vi "GRAPH.vi"() -> ()   [LabVIEW 2013]
panel:
  in  "Power":i32 min=0 max=100 step=1
  out "Waveform Chart":i32(graph)
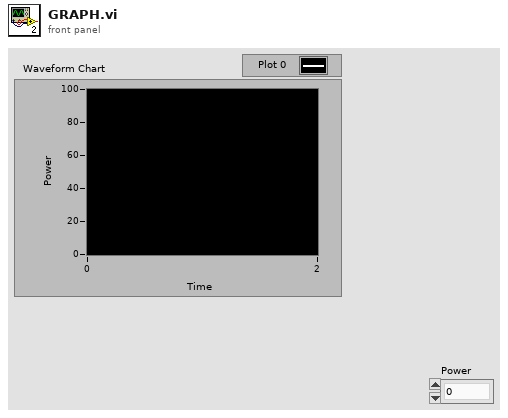
[diagram p1: front panel]
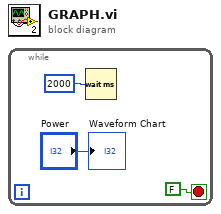
[diagram p0: block diagram]
diagram:
  n1 = while {
    stop <- FALSE stop-if-true
    n2 = Wait (ms)(milliseconds to wait=u32 2000 ("millisecond timer value")) -> ()  [unwired: 1 out]
    "Waveform Chart" <- "Power"
  }
